vi "Setup_zurichInst.vi"(8 "error in (no error)":errorcluster, 11 "Handle In":T1 {"Handle" format="0x%08x"; "Conn" format="0x%08x"}) -> (0 "error out":errorcluster, 3 "Handle Out":T1 {"Handle" format="0x%08x"; "Conn" format="0x%08x"})   [LabVIEW 2019]
uses:
  Equipment/Zurich Instruments LabOne/Public/ziTypeHandle.ctl
  Instrument_Setup.vi
  Equipment/Zurich Instruments LabOne/Public/Configure/ziSetValueDouble.vi
  Equipment/Zurich Instruments LabOne/Zurich Instruments LabOne.lvlib
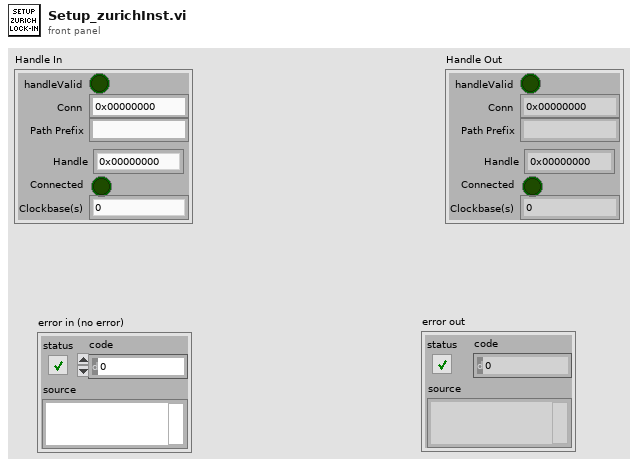
[diagram p1: front panel]
types:
  T1 = typedef "Zurich Instruments LabOne.lvlib/ziTypeHandle.ctl" = cluster{"handleValid":bool, "Conn":u64, "Path Prefix":string, "Handle":u64, "Connected":bool, "Clockbase(s)":dbl}
  T2 = cluster{"Adress":string, "Load Settings from File":bool, "Output_Demod1":enum16{"Aux 1", "Aux 2", "Aux 3", "Aux 4"}, "Input_Demod1":enum16{"Sig In 1", "Curr In 1", "Trigger 1", "Trigger 2", "Aux Out 1", "Aux Out 2", "Aux Out 3", "Aux Out 4", "Aux In 1", "Aux In 2", "Constant"}, "Input_Mode_Demod1":enum16{"single ended", "differential"}, "Bandwith_Mode_Demod1":enum16{"TC", "BW NEP", "BW 3dB"}, "Bandw_Value_demod1":dbl, "Demod1_Range":dbl, "Demod1_Harmonic":dbl, "Trigger_Demod1":enum16{"Manual", "External"}, "osc1_freq":dbl, "osc1_amp":dbl, "Demod1_scaling":dbl, "osc2_freq":dbl, "osc2_amp":dbl, "osc3_freq":dbl, "osc3_amp":dbl, "osc4_freq":dbl, "osc4_amp":dbl, "Demod1_Phase (deg)":dbl, "Demod1_order":ext, "Demod1_coupling":enum16{"DC", "AC"}, "Demod1_shields":enum16{"Ground", "Float"}, "Demod1_input_resistance":enum16{"10M", "50"}, "Demod1_Ref_oscillator":ext, "Demod1_output_imp":enum16{"Disable", "Enable"}, "Demod1_output_diff":enum16{"Disable", "Enable"}, "Demod1_rate":dbl, "Demod1_Output_range":dbl, "Output_Demod2":enum16{"Aux 1", "Aux 2", "Aux 3", "Aux 4"}, "Demod2_input":enum16{"Sig In 1", "Curr In 1", "Trigger 1", "Trigger 2", "Aux Out 1", "Aux Out 2", "Aux Out 3", "Aux Out 4", "Aux In 1", "Aux In 2", "Constant"}, "Input_Mode_Demod2":enum16{"single ended", "differential"}, "Bandwith_Mode_Demod2":enum16{"TC", "BW NEP", "BW 3dB"}, "Bandw_Value_demod2":dbl, "Demod2_Range":dbl, "Demod2_Harmonic":dbl, "Trigger_Demod2":enum16{"Manual", "External"}, "Demod2_scaling":dbl, "Demod2_Phase (deg)":dbl, "Demod2_order":ext, "Demod2_coupling":enum16{"DC", "AC"}, "Demod2_shields":enum16{"Ground", "Float"}, "Demod2_input_resistance":enum16{"10M", "50"}, "Demod2_Ref_oscillator":ext, "Demod2_output_imp":enum16{"Disable", "Enable"}, "Demod2_output_diff":enum16{"Disable", "Enable"}, "Demod2_rate":dbl, "Demod2_Output_range":dbl, "Output_Demod3":enum16{"Aux 1", "Aux 2", "Aux 3", "Aux 4"}, "Demod3_input":enum16{"Sig In 1", "Curr In 1", "Trigger 1", "Trigger 2", "Aux Out 1", "Aux Out 2", "Aux Out 3", "Aux Out 4", "Aux In 1", "Aux In 2", "Constant"}, "Input_Mode_Demod3":enum16{"single ended", "differential"}, "Bandwith_Mode_Demod2":enum16{"TC", "BW NEP", "BW 3dB"}, "Bandw_Value_demod3":dbl, "Demod3_Range":dbl, "Demod3_Harmonic":dbl, "Trigger_Demod3":enum16{"Manual", "External"}, "Demod3_scaling":dbl, "Demod3_Phase (deg)":dbl, "Demod3_order":ext, "Demod3_coupling":enum16{"DC", "AC"}, "Demod3_shields":enum16{"Ground", "Float"}, "Demod3_input_resistance":enum16{"10M", "50"}, "Demod3_Ref_oscillator":ext, "Demod3_output_imp":enum16{"Disable", "Enable"}, "Demod3_output_diff":enum16{"Disable", "Enable"}, "Demod3_rate":dbl, "Demod3_Output_range":dbl, "Output_Demod4":enum16{"Aux 1", "Aux 2", "Aux 3", "Aux 4"}, "Demod4_input":enum16{"Sig In 1", "Curr In 1", "Trigger 1", "Trigger 2", "Aux Out 1", "Aux Out 2", "Aux Out 3", "Aux Out 4", "Aux In 1", "Aux In 2", "Constant"}, "Input_Mode_Demod4":enum16{"single ended", "differential"}, "Bandwith_Mode_Demod4":enum16{"TC", "BW NEP", "BW 3dB"}, "Bandw_Value_demod4":dbl, "Demod4_Range":dbl, "Demod4_Harmonic":dbl, "Trigger_Demod4":enum16{"Manual", "External"}, "Demod4_scaling":dbl, "Demod4_Phase (deg)":dbl, "Demod4_order":ext, "Demod4_coupling":enum16{"DC", "AC"}, "Demod4_shields":enum16{"Ground", "Float"}, "Demod4_input_resistance":enum16{"10M", "50"}, "Demod4_Ref_oscillator":ext, "Demod4_output_imp":enum16{"Disable", "Enable"}, "Demod4_output_diff":enum16{"Disable", "Enable"}, "Demod4_rate":dbl, "Demod4_Output_range":dbl, "Oscillator1_Amp_units":enum16{"Vpk", "Vrms", "VdBm"}, "Oscillator4_Amp_units":enum16{"Vpk", "Vrms", "VdBm"}, "Oscillator2_Amp_units":enum16{"Vpk", "Vrms", "VdBm"}, "Oscillator3_Amp_units":enum16{"Vpk", "Vrms", "VdBm"}, "Demod1_sync_filter":enum16{"Disable", "Enable"}, "Demod 1 (on/off)":bool, "Demod 2 (on/off) ":bool, "Demod 3 (on/off) ":bool, "Demod 4 (on/off) ":bool, " Sigouts 1 (on/off)":bool, " Sigouts 2 (on/off) ":bool, " Sigouts 3 (on/off)":bool, " Sigouts 4 (on/off) ":bool, "Demod2_sync_filter":enum16{"Disable", "Enable"}, "Demod1_auto_outp_rang":enum16{"Disable", "Enable"}, "Demod2_auto_outp_rang ":enum16{"Disable", "Enable"}}
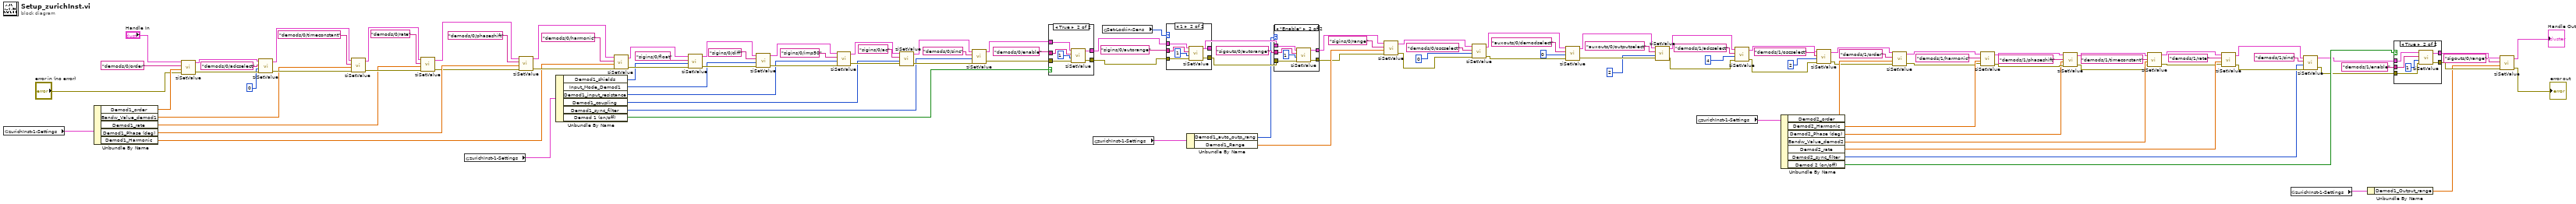
[diagram p0: block diagram]
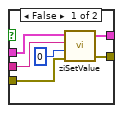
[diagram p2: hidden frame]
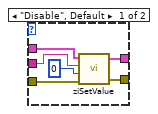
[diagram p3: hidden frame]
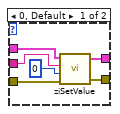
[diagram p4: hidden frame]
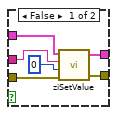
[diagram p5: hidden frame]
diagram:
  n1 = global read "Instrument_Setup.vi" "zurichInst-1-Settings"() -> (w86:T2)
  n2 = Unbundle By Name(w86) -> ("Demod1_order"=w85:ext, "Bandw_Value_demod1"=w84:dbl, "Demod1_rate"=w83:dbl, "Demod1_Phase (deg)"=w82:dbl, "Demod1_Harmonic"=w81:dbl)
  n3 = call-poly "ziSetValue.vi"("Error In"="error in (no error)", "Value"=w85, "Path"="demods/0/order", "Handle In"="Handle In") -> ("Error Out"=w117:errorcluster, "Handle Out"=w118:T1)  [unwired: 1 in]
  n4 = call-poly "ziSetValue.vi"("Error In"=w117, "Value"=0, "Path"="demods/0/adcselect", "Handle In"=w118) -> ("Error Out"=w116:errorcluster, "Handle Out"=w115:T1)  [unwired: 1 in]
  n5 = call-poly "ziSetValue.vi"("Error In"=w116, "Value"=w84, "Path"="demods/0/timeconstant", "Handle In"=w115) -> ("Error Out"=w113:errorcluster, "Handle Out"=w114:T1)  [unwired: 1 in]
  n6 = call-poly "ziSetValue.vi"("Error In"=w113, "Value"=w83, "Path"="demods/0/rate", "Handle In"=w114) -> ("Error Out"=w71:errorcluster, "Handle Out"=w70:T1)  [unwired: 1 in]
  n7 = global read "Instrument_Setup.vi" "zurichInst-1-Settings"() -> (w80:T2)
  n8 = call-poly "ziSetValue.vi"("Error In"=w71, "Value"=w82, "Path"="demods/0/phaseshift", "Handle In"=w70) -> ("Error Out"=w112:errorcluster, "Handle Out"=w111:T1)  [unwired: 1 in]
  n9 = Unbundle By Name(w80) -> ("Demod1_shields"=w79:enum16{"Ground", "Float"}, "Input_Mode_Demod1"=w78:enum16{"single ended", "differential"}, "Demod1_input_resistance"=w77:enum16{"10M", "50"}, "Demod1_coupling"=w76:enum16{"DC", "AC"}, "Demod1_sync_filter"=w75:enum16{"Disable", "Enable"}, "Demod 1 (on/off)"=w74:bool)
  n10 = call-poly "ziSetValue.vi"("Error In"=w112, "Value"=w81, "Path"="demods/0/harmonic", "Handle In"=w111) -> ("Error Out"=w105:errorcluster, "Handle Out"=w103:T1)  [unwired: 1 in]
  n11 = call-poly "ziSetValue.vi"("Error In"=w105, "Value"=w79, "Path"="sigins/0/float", "Handle In"=w103) -> ("Error Out"=w102:errorcluster, "Handle Out"=w101:T1)  [unwired: 1 in]
  n12 = call-poly "ziSetValue.vi"("Error In"=w102, "Value"=w78, "Path"="sigins/0/diff", "Handle In"=w101) -> ("Error Out"=w99:errorcluster, "Handle Out"=w98:T1)  [unwired: 1 in]
  n13 = call-poly "ziSetValue.vi"("Error In"=w99, "Value"=w77, "Path"="sigins/0/imp50", "Handle In"=w98) -> ("Error Out"=w96:errorcluster, "Handle Out"=w95:T1)  [unwired: 1 in]
  n14 = call-poly "ziSetValue.vi"("Error In"=w96, "Value"=w76, "Path"="sigins/0/ac", "Handle In"=w95) -> ("Error Out"=w93:errorcluster, "Handle Out"=w92:T1)  [unwired: 1 in]
  n15 = call-poly "ziSetValue.vi"("Error In"=w93, "Value"=w75, "Path"="demods/0/sinc", "Handle In"=w92) -> ("Error Out"=w90:errorcluster, "Handle Out"=w89:T1)  [unwired: 1 in]
  n16 = case shown="True" w74 {
    tunnel: w90 -> [w124 w131]
    tunnel: w89 -> [w123 w130]
    tunnel: [w121 w129] -> w68
    tunnel: [w122 w128] -> w69
    tunnel: "demods/0/enable" -> [w125 w127]
    frame False {
      n17 = call-poly "ziSetValue.vi"("Error In"=w124, "Value"=0, "Path"=w125, "Handle In"=w123) -> ("Error Out"=w121:errorcluster, "Handle Out"=w122:T1)  [unwired: 1 in]
    }
    frame True {
      n18 = call-poly "ziSetValue.vi"("Error In"=w131, "Value"=1, "Path"=w127, "Handle In"=w130) -> ("Error Out"=w129:errorcluster, "Handle Out"=w128:T1)  [unwired: 1 in]
    }
  }
  n19 = global read "Instrument_Setup.vi" "zurichInst-1-Settings"() -> (w65:T2)
  n20 = global read "Instrument_Setup.vi" "Set-Lockin-Sens"() -> (w67:u16)
  n21 = case shown="1" w67 {
    tunnel: w69 -> [w137 w143]
    tunnel: "sigins/0/autorange" -> [w133 w142]
    tunnel: [w136 w140] -> w64
    tunnel: [w135 w139] -> w63
    tunnel: w68 -> [w134 w138]
    frame 0, Default {
      n22 = call-poly "ziSetValue.vi"("Error In"=w134, "Value"=0, "Path"=w133, "Handle In"=w137) -> ("Error Out"=w135:errorcluster, "Handle Out"=w136:T1)  [unwired: 1 in]
    }
    frame 1 {
      n23 = call-poly "ziSetValue.vi"("Error In"=w138, "Value"=1, "Path"=w142, "Handle In"=w143) -> ("Error Out"=w139:errorcluster, "Handle Out"=w140:T1)  [unwired: 1 in]
    }
  }
  n24 = Unbundle By Name(w65) -> ("Demod1_auto_outp_rang"=w61:enum16{"Disable", "Enable"}, "Demod1_Range"=w60:dbl)
  n25 = case shown="\"Enable\"" w61 {
    tunnel: w64 -> [w149 w155]
    tunnel: "sigouts/0/autorange" -> [w145 w154]
    tunnel: [w148 w152] -> w54
    tunnel: [w147 w151] -> w53
    tunnel: w63 -> [w146 w150]
    frame "Disable", Default {
      n26 = call-poly "ziSetValue.vi"("Error In"=w146, "Value"=0, "Path"=w145, "Handle In"=w149) -> ("Error Out"=w147:errorcluster, "Handle Out"=w148:T1)  [unwired: 1 in]
    }
    frame "Enable" {
      n27 = call-poly "ziSetValue.vi"("Error In"=w150, "Value"=1, "Path"=w154, "Handle In"=w155) -> ("Error Out"=w151:errorcluster, "Handle Out"=w152:T1)  [unwired: 1 in]
    }
  }
  n28 = call-poly "ziSetValue.vi"("Error In"=w53, "Value"=w60, "Path"="sigins/0/range", "Handle In"=w54) -> ("Error Out"=w56:errorcluster, "Handle Out"=w57:T1)  [unwired: 1 in]
  n29 = call-poly "ziSetValue.vi"("Error In"=w56, "Value"=0, "Path"="demods/0/oscselect", "Handle In"=w57) -> ("Error Out"=w51:errorcluster, "Handle Out"=w50:T1)  [unwired: 1 in]
  n30 = call-poly "ziSetValue.vi"("Error In"=w51, "Value"=0, "Path"="auxouts/0/demodselect", "Handle In"=w50) -> ("Error Out"=w47:errorcluster, "Handle Out"=w48:T1)  [unwired: 1 in]
  n31 = call-poly "ziSetValue.vi"("Error In"=w47, "Value"=2, "Path"="auxouts/0/outputselect", "Handle In"=w48) -> ("Error Out"=w43:errorcluster, "Handle Out"=w44:T1)  [unwired: 1 in]
  n32 = global read "Instrument_Setup.vi" "zurichInst-1-Settings"() -> (w36:T2)
  n33 = call-poly "ziSetValue.vi"("Error In"=w43, "Value"=4, "Path"="demods/1/adcselect", "Handle In"=w44) -> ("Error Out"=w38:errorcluster, "Handle Out"=w37:T1)  [unwired: 1 in]
  n34 = Unbundle By Name(w36) -> ("Demod2_order"=w34:ext, "Demod2_Harmonic"=w30:dbl, "Demod2_Phase (deg)"=w24:dbl, "Bandw_Value_demod2"=w22:dbl, "Demod2_rate"=w17:dbl, "Demod2_sync_filter"=w12:enum16{"Disable", "Enable"}, "Demod 2 (on/off)"=w10:bool)
  n35 = call-poly "ziSetValue.vi"("Error In"=w38, "Value"=2, "Path"="demods/1/oscselect", "Handle In"=w37) -> ("Error Out"=w33:errorcluster, "Handle Out"=w32:T1)  [unwired: 1 in]
  n36 = call-poly "ziSetValue.vi"("Error In"=w33, "Value"=w34, "Path"="demods/1/order", "Handle In"=w32) -> ("Error Out"=w29:errorcluster, "Handle Out"=w28:T1)  [unwired: 1 in]
  n37 = call-poly "ziSetValue.vi"("Error In"=w29, "Value"=w30, "Path"="demods/1/harmonic", "Handle In"=w28) -> ("Error Out"=w25:errorcluster, "Handle Out"=w26:T1)  [unwired: 1 in]
  n38 = call-poly "ziSetValue.vi"("Error In"=w25, "Value"=w24, "Path"="demods/1/phaseshift", "Handle In"=w26) -> ("Error Out"=w21:errorcluster, "Handle Out"=w20:T1)  [unwired: 1 in]
  n39 = call-poly "ziSetValue.vi"("Error In"=w21, "Value"=w22, "Path"="demods/1/timeconstant", "Handle In"=w20) -> ("Error Out"=w16:errorcluster, "Handle Out"=w18:T1)  [unwired: 1 in]
  n40 = call-poly "ziSetValue.vi"("Error In"=w16, "Value"=w17, "Path"="demods/1/rate", "Handle In"=w18) -> ("Error Out"=w13:errorcluster, "Handle Out"=w14:T1)  [unwired: 1 in]
  n41 = global read "Instrument_Setup.vi" "zurichInst-1-Settings"() -> (w4:T2)
  n42 = call-poly "ziSetValue.vi"("Error In"=w13, "Value"=w12, "Path"="demods/1/sinc", "Handle In"=w14) -> ("Error Out"=w8:errorcluster, "Handle Out"=w9:T1)  [unwired: 1 in]
  n43 = Unbundle By Name(w4) -> ("Demod1_Output_range"=w3:dbl)
  n44 = case shown="True" w10 {
    tunnel: w8 -> [w160 w167]
    tunnel: w9 -> [w159 w166]
    tunnel: [w157 w165] -> w5
    tunnel: [w158 w164] -> w7
    tunnel: "demods/1/enable" -> [w161 w163]
    frame False {
      n45 = call-poly "ziSetValue.vi"("Error In"=w160, "Value"=0, "Path"=w161, "Handle In"=w159) -> ("Error Out"=w157:errorcluster, "Handle Out"=w158:T1)  [unwired: 1 in]
    }
    frame True {
      n46 = call-poly "ziSetValue.vi"("Error In"=w167, "Value"=1, "Path"=w163, "Handle In"=w166) -> ("Error Out"=w165:errorcluster, "Handle Out"=w164:T1)  [unwired: 1 in]
    }
  }
  n47 = call-poly "ziSetValue.vi"("Error In"=w5, "Value"=w3, "Path"="sigouts/0/range", "Handle In"=w7) -> ("Error Out"=→"error out":errorcluster, "Handle Out"=→"Handle Out":T1)  [unwired: 1 in]
